vi "Connect SCSI Passthrough.vi"(8 "error in (no error)":errorcluster, 10 "Product":string="MEMS Tester     \u0000", 11 "Vendor":string="ALU     \u0000") -> (0 "error out":errorcluster)   [LabVIEW 2014]
uses:
  BasicDLL.dll
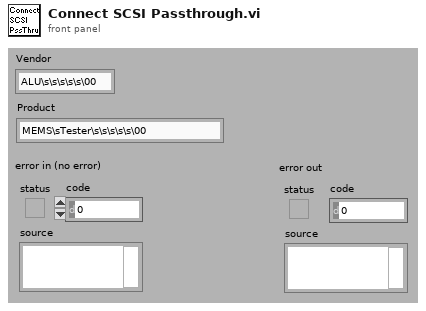
[diagram p1: front panel]
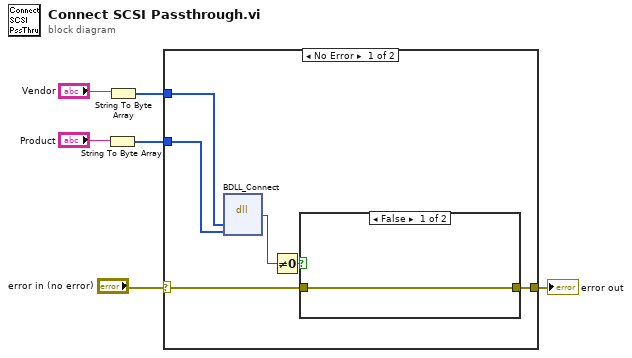
[diagram p0: block diagram]
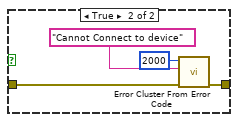
[diagram p2: hidden frame]
diagram:
  n1 = String To Byte Array(string="Product") -> (unsigned byte array=w3:u8[])
  n2 = String To Byte Array(string="Vendor") -> (unsigned byte array=w4:u8[])
  n3 = case shown="No Error" "error in (no error)" {
    selector: "error in (no error)" -> [w7 w18]
    tunnel: w4 -> [w12 _]
    tunnel: w3 -> [w11 _]
    tunnel: [w10 w18] -> w2
    frame No Error {
      n4 = dll-call lib="C:/Users/SingleCell/Desktop/Biostinger/BioStingerGUI/Gener8 Software/Low Level USB/Low Level USB/BasicDLL.dll" fn="BDLL_Connect"("product"=w12, "vendor"=w11) -> (w8:i32)  [unwired: 5 in, 2 out]
      n5 = Not Equal To 0?(x=w8) -> (x != 0?=w9:bool)
      n6 = case shown="False" w9 {
        tunnel: [w13 w17] -> w10
        tunnel: w7 -> [w13 w16]
        frame False {
        }
        frame True {
          n7 = call <vilib>:"Error Cluster From Error Code.vi"("error in (no error)"=w16, "error message (\"\")"="Cannot Connect to device" ("error message (\"\")"), "error code (0)"=2000) -> ("error out"=w17:errorcluster)  [unwired: 6 in]
        }
      }
    }
    frame Error {
    }
  }
  "error out" <- w2
